vi "DiffDriveTrainSim_ClampInput.vi"(9 "BatteryVoltage":dbl, 11 "U":T1) -> (3 "Normalized U":T1)   [LabVIEW 2019, in "Trajectory_Library.lvlib"]
doc: "Creates a new LINEAR SYSTEM data cluster with the specified values. \n\n\nInputs: \n - XXX -- XXX.\n\nOutputs:\n - XXX -- XXX."
uses:
  <vilib>/Analysis/Matrix/Datatypes/RealMatrix.ctl
  MatBuilder_Create.vi
  Trajectory_Library.lvlib
  <vilib>/Analysis/Matrix/NI_Matrix.lvlib
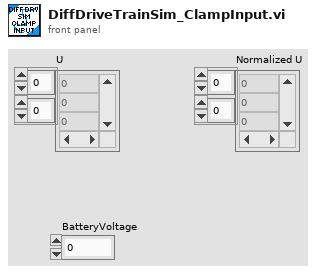
[diagram p1: front panel]
types:
  T1 = typedef "NI_Matrix.lvlib/RealMatrix.ctl" = dbl[][]
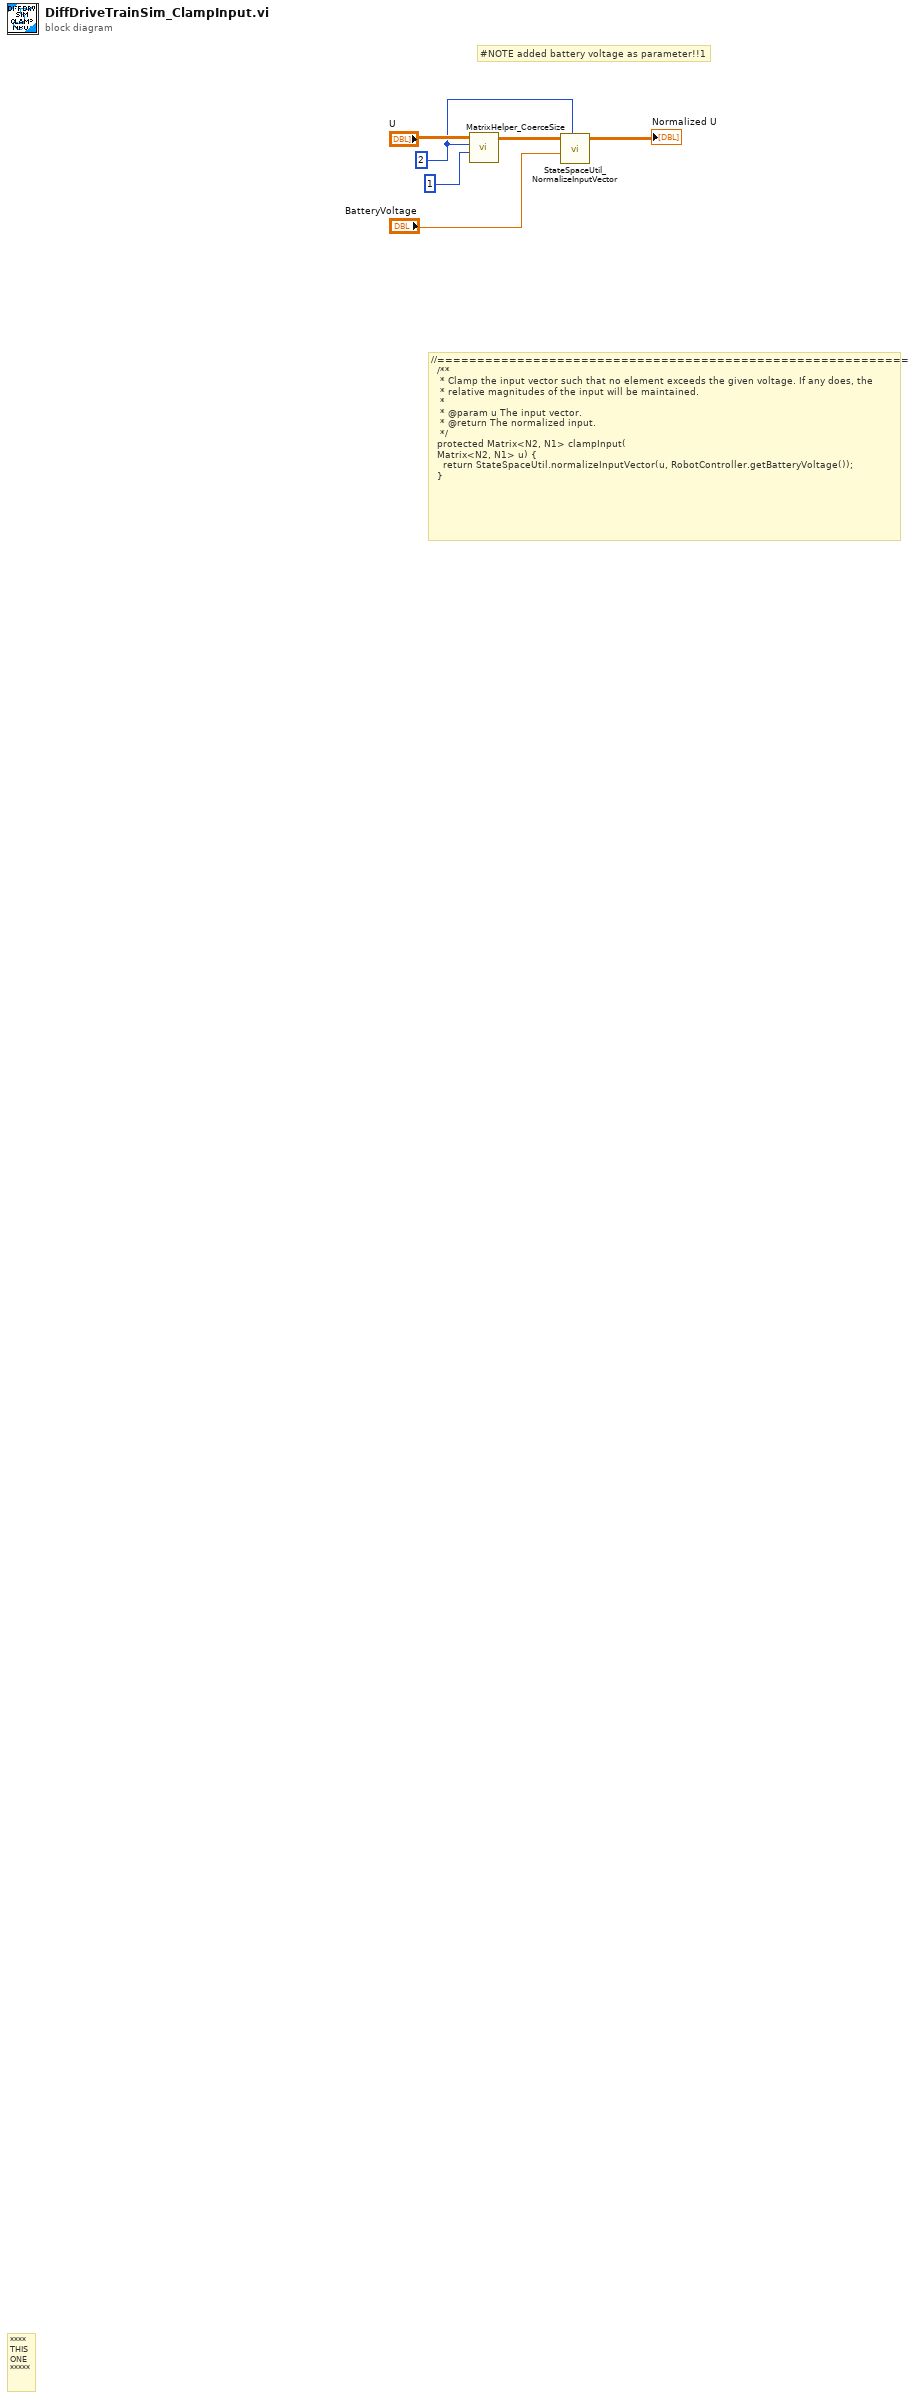
[diagram p0: block diagram]
diagram:
  w4 = 2 ("Rows")
  # "//============================================================\n  /**\n   * Clamp the input vector such that no element exceeds the given voltage. If any does, the\n   * relative magnitudes of the input will be maintained.\n   *\n   * @param u The input vector.\n   * @return The normalized input.\n   */\n  protected Matrix<N2, N1> clampInput(\n\t\tMatrix<N2, N1> u) {\n    return StateSpaceUtil.normalizeInputVector(u, RobotController.getBatteryVoltage());\n  }"
  # "#NOTE added battery voltage as parameter!!1"
  # "****\nTHIS\nONE\n*****"
  n1 = call "MatrixHelper_CoerceSize.vi"("Columns"=1, "Rows"=w4, "input matrix"="U") -> ("output matrix"=w3:T1)  [unwired: 8 in]
  n2 = call "StateSpaceUtil_NormalizeInputVector.vi"("J"=w4, "Max_Magnitude"="BatteryVoltage", "U"=w3) -> ("NormalizedU"=→"Normalized U":T1)  [unwired: 8 in]
